vi "F Dwf Digital In Trigger Info.vi"(0 "hdwf":i32, 1 "pfsEdgeFall":u32, 5 "pfsLevelLow":u32, 7 "pfsLevelHigh":u32, 9 "pfsEdgeRise":u32, 11 "error in (no error)":errorcluster) -> (3 "pfsEdgeFall out":u32, 4 "function return":i32, 6 "pfsLevelLow out":u32, 8 "pfsLevelHigh out":u32, 10 "pfsEdgeRise out":u32, 15 "error out":errorcluster)   [LabVIEW 2019, in "Olasdwf.lvlib"]
doc: "DWFAPI int FDwfDigitalInTriggerInfo(HDWF hdwf, unsigned int *pfsLevelLow, unsigned int *pfsLevelHigh, unsigned int *pfsEdgeRise, unsigned int *pfsEdgeFall);"
uses:
  Olasdwf.lvlib
  Windows/System32/dwf.dll
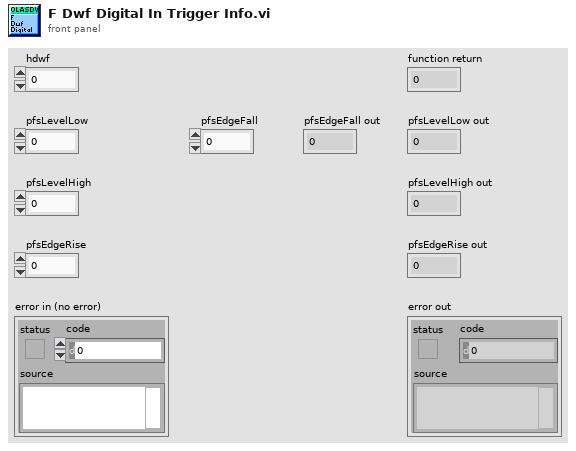
[diagram p1: front panel]
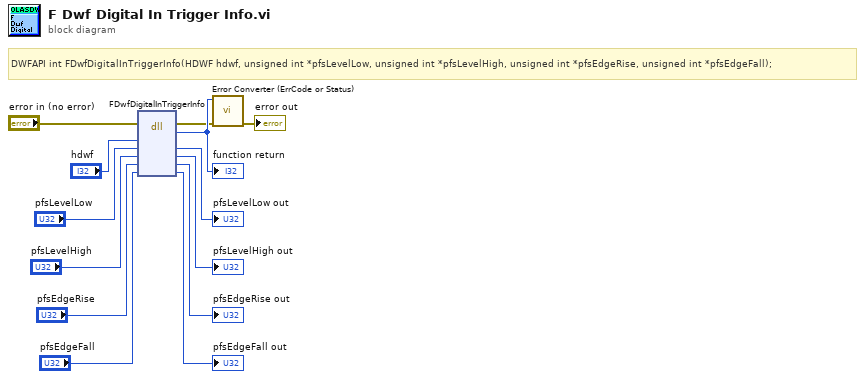
[diagram p0: block diagram]
diagram:
  # "DWFAPI int FDwfDigitalInTriggerInfo(HDWF hdwf, unsigned int *pfsLevelLow, unsigned int *pfsLevelHigh, unsigned int *pfsEdgeRise, unsigned int *pfsEdgeFall);"
  n1 = dll-call lib="C:/Windows/System32/dwf.*" fn="FDwfDigitalInTriggerInfo"(error in="error in (no error)", "hdwf"="hdwf", "pfsLevelLow"="pfsLevelLow", "pfsLevelHigh"="pfsLevelHigh", "pfsEdgeRise"="pfsEdgeRise", "pfsEdgeFall"="pfsEdgeFall") -> (error out=w2:errorcluster, w13:i32, "pfsLevelLow"=→"pfsLevelLow out":u32, "pfsLevelHigh"=→"pfsLevelHigh out":u32, "pfsEdgeRise"=→"pfsEdgeRise out":u32, "pfsEdgeFall"=→"pfsEdgeFall out":u32)  [unwired: 3 in, 1 out]
  "function return" <- w13
  n2 = call "Error Converter (ErrCode or Status).vi"("error in (no error)"=w2, "error code"=w13) -> ("error out"=→"error out":errorcluster)  [unwired: 9 in]
